vi "GrabBackground.vi"() -> ()   [LabVIEW 2011]
uses:
  <vilib>/vision/Image Controls.llb/IMAQ Image.ctl
  Main/Camera/CIGrabParams.ctl
  qtrk/QTrkLVBinding/QTrkInstance.ctl
  qtrk/QTrkLVBinding/ResultManagerInstance.ctl
  Main/Camera/CIGrabControlMsg.ctl
  Main/Camera/CIGrabControlMsgEnum.ctl
  Main/GlobalVariables.vi
  <vilib>/vision/NI_Vision_Development_Module.lvlib
panel:
  out "Image-Background":T1(plugin-control)
  in  "Export path":path
  in  "F_a":sgl=0.002
  in  "Save":bool
  out "Tmp Img":T1
  out "Background":T1(plugin-control)
  in  "Grab loop":bool
  out "Frame #":i32
  out "Image":T1(plugin-control)
  in  "Grab Framerate (Hz)":i32=20
  in  "Grab background":bool
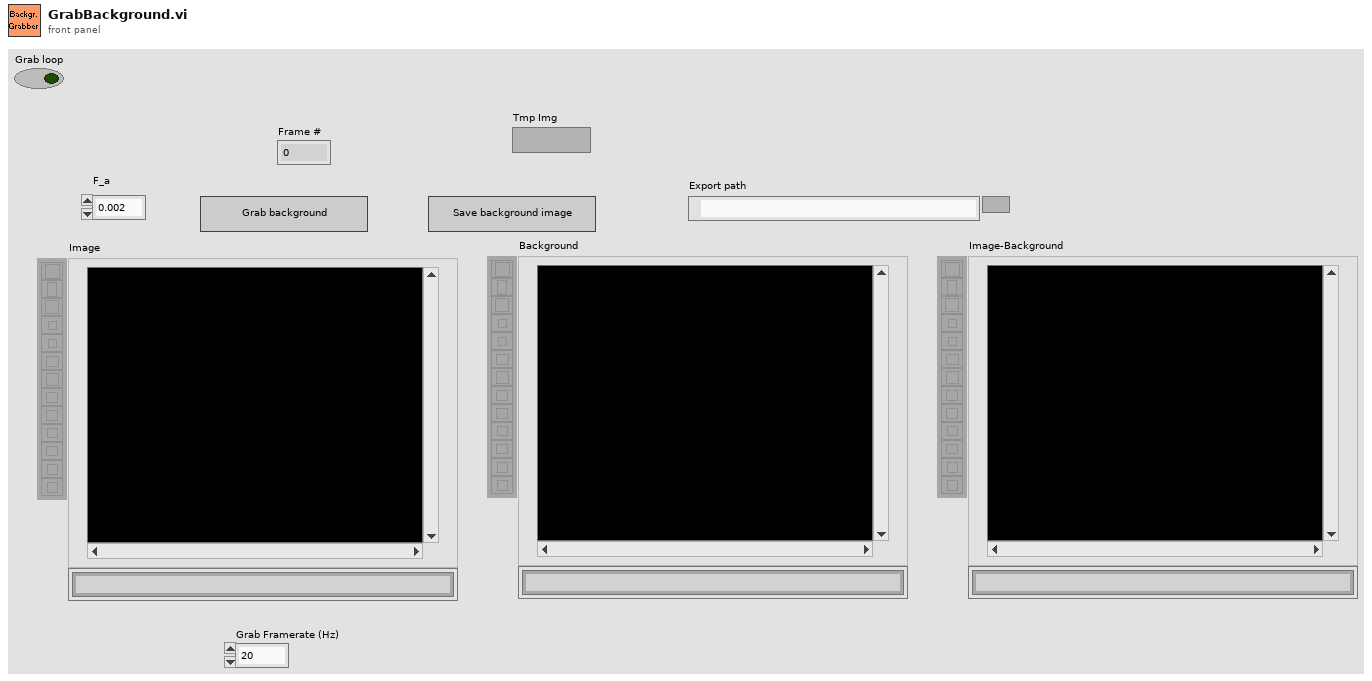
[diagram p1: front panel]
types:
  T1 = typedef "IMAQ Image.ctl" = refnum<image>
  T2 = typedef "Image Type" = u32
  T3 = enum16{"big-endian, network order", "native, host order", "little-endian"}
  T4 = typedef "CIGrabParams.ctl" = cluster{"QTrk Instance":T5, "ResultManager":T6, "Send to queue?":bool, "Force full-frame capture":bool}
  T5 = typedef "QTrkInstance.ctl" = cluster{"QTrk Pointer":u64}
  T6 = typedef "ResultManagerInstance.ctl" = cluster{"InstancePtr":u64}
  T7 = typedef "CIGrabControlMsg.ctl" = cluster{"Msg":T8}
  T8 = typedef "CIGrabControlMsgEnum.ctl" = enum16{"Stop", "EnableTracking", "DisableTracking"}
  T9 = typedef "CIGrabType.ctl" = refnum<vi>
  T10 = typedef "CmdData_NewFrame.ctl" = cluster{"Buffer Image":T1, "Frame #":i32, "Hardware ROI Index":i32, "Timestamp":dbl, "Type":T11}
  T11 = typedef "CmdEnum_CameraFrameType.ctl" = enum16{"Full", "HardwareROI", "EndGrabMarker"}
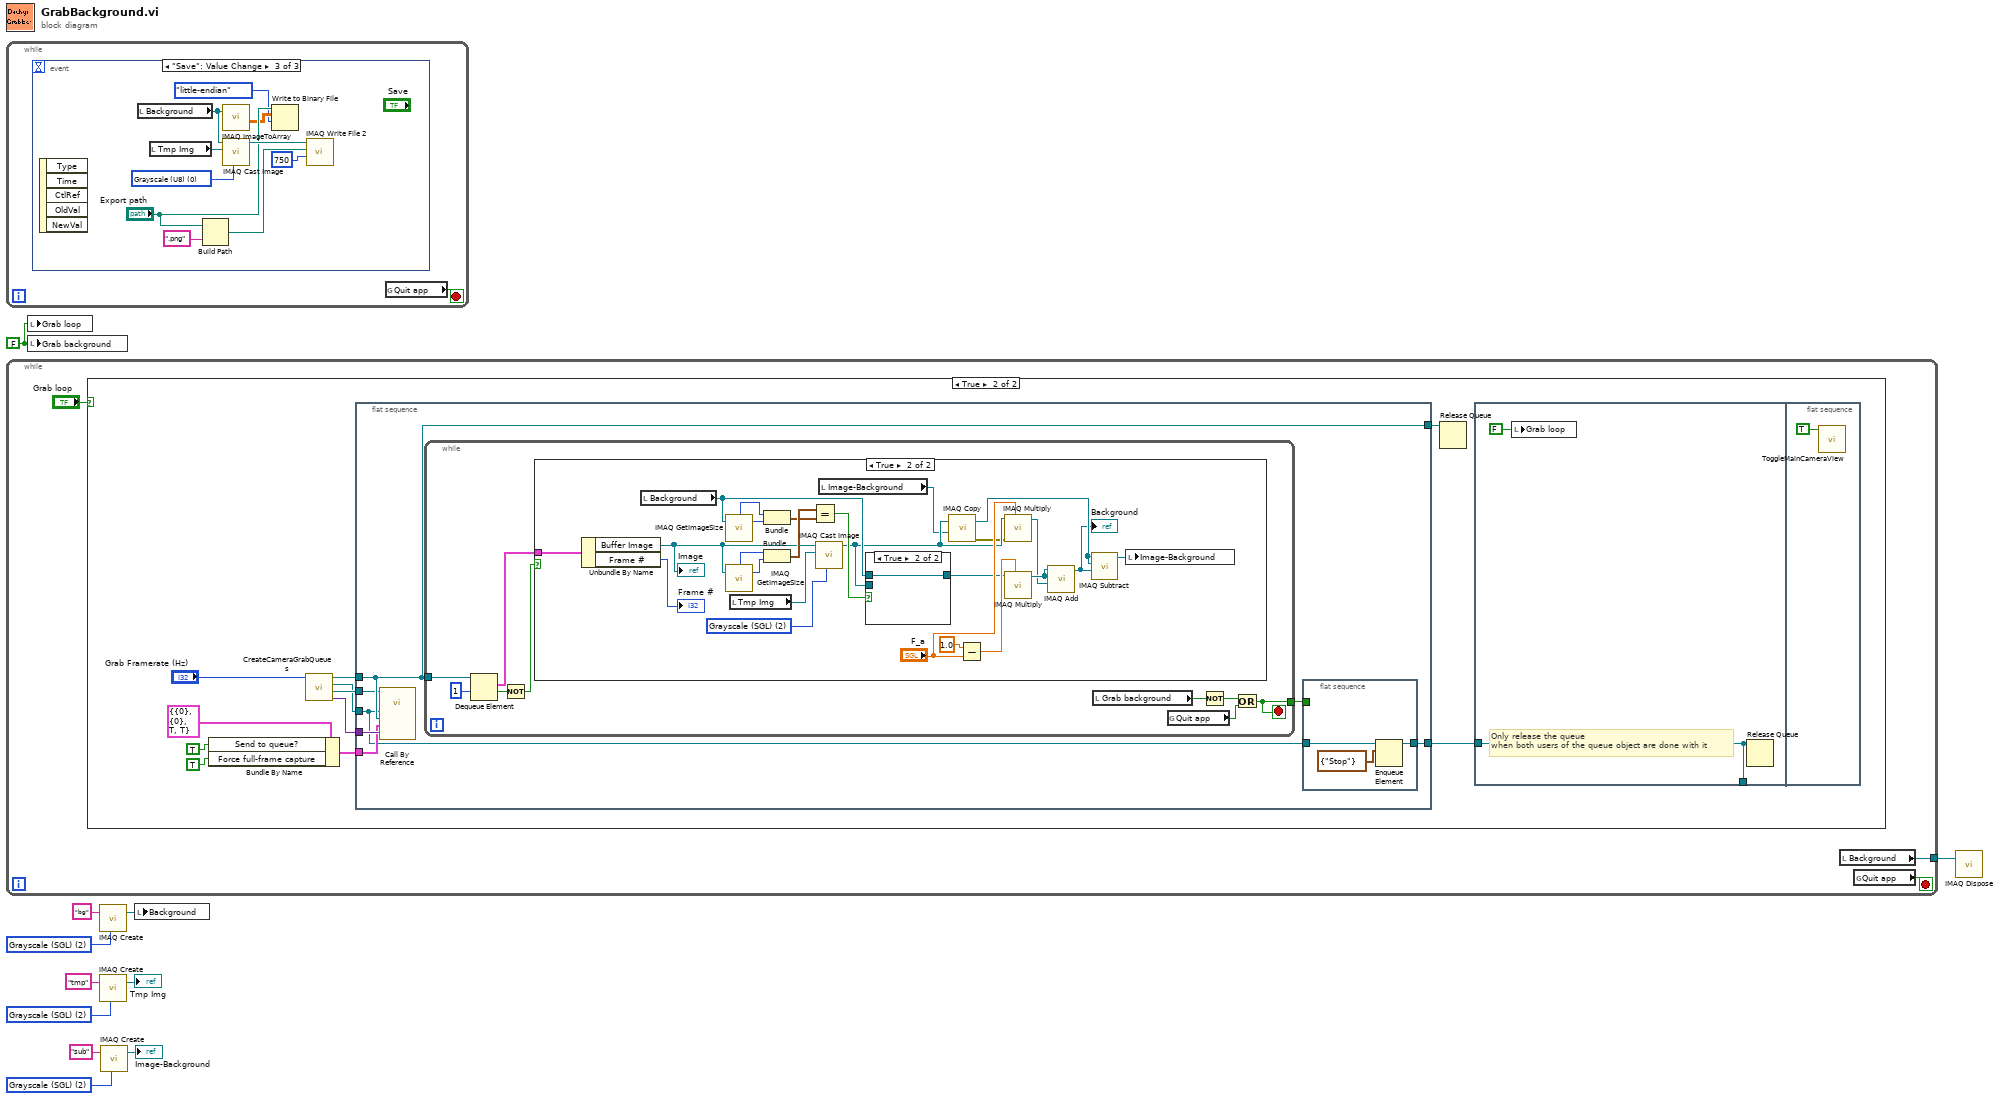
[diagram p0: block diagram]
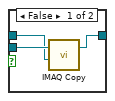
[diagram p4: hidden frame]
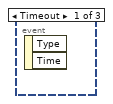
[diagram p5: hidden frame]
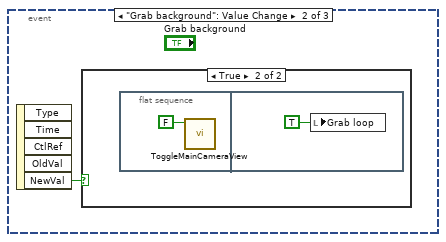
[diagram p6: hidden frame]
diagram:
  w3 = T2 2 items=["Grayscale (U8)", "Grayscale (I16)", "Grayscale (SGL)", "Complex (CSG)", "RGB (U32)", "HSL (U32)", "RGB (U64)", "Grayscale (U16)"] ("Image Type")
  w4 = T2 2 items=["Grayscale (U8)", "Grayscale (I16)", "Grayscale (SGL)", "Complex (CSG)", "RGB (U32)", "HSL (U32)", "RGB (U64)", "Grayscale (U16)"] ("Image Type")
  w5 = T2 2 items=["Grayscale (U8)", "Grayscale (I16)", "Grayscale (SGL)", "Complex (CSG)", "RGB (U32)", "HSL (U32)", "RGB (U64)", "Grayscale (U16)"] ("Image Type")
  w11 = FALSE ("Grab background")
  n1 = while {
    stop <- w12 stop-if-true
    n2 = event shown="[2] \"Save\": Value Change" {
      selector: _ -> [_ _ _]
      dyn-events: _ -> [_ _ _]
      timeout: _ -> [_ _ _]
      event Timeout {
        n3 = event-data() -> ()  [unwired: 1 in, 2 out]
      }
      event "Grab background": Value Change {
        n4 = event-data() -> ("NewVal"=w13:bool)  [unwired: 1 in, 4 out]
        n5 = case shown="True" w13 {
          frame False {
          }
          frame True {
            n6 = flat-sequence {
              frame #0 {
                n7 = call "ToggleMainCameraView.vi"("Enable? (T)"=FALSE) -> ()  [unwired: 11 in]
              }
              frame #1 {
                n8 = local write "Grab loop"(TRUE ("Grab loop")) -> ()
              }
            }
          }
        }
      }
      event "Save": Value Change {
        w22 = T2 0 items=["Grayscale (U8)", "Grayscale (I16)", "Grayscale (SGL)", "Complex (CSG)", "RGB (U32)", "HSL (U32)", "RGB (U64)", "Grayscale (U16)"] ("Image Type")
        n9 = event-data() -> ()  [unwired: 1 in, 5 out]
        n10 = local read "Background"() -> (w20:T1)
        n11 = local read "Tmp Img"() -> (w23:T1)
        n12 = Build Path(base path="Export path", name or relative path=".png") -> (appended path=w16:path)
        n13 = call "IMAQ ImageToArray"("Image"=w20) -> ("Image Pixels (Float)"=w18:sgl[][])  [unwired: 3 in, 4 out]
        n14 = call "IMAQ Cast Image"("Image Type"=w22, "Image Dst"=w23, "Image Src"=w20) -> ("Image Dst Out"=w21:T1)  [unwired: 7 in, 1 out]
        n15 = Write to Binary File(file (use dialog)="Export path", data=w18, 9:T3."little-endian" ("byte order (0:big-endian, network order)")) -> ()  [unwired: 3 in, 3 out]
        n16 = call-poly "IMAQ Write File 2"("Image Quality"=u32 750, "File Path"=w16, "Image"=w21) -> ()  [unwired: 7 in, 2 out]
      }
    }
    n17 = global read "GlobalVariables.vi" "Quit app"() -> (w12:bool)
  }
  n18 = while {
    tunnel: [w26] -> w8
    stop <- w28 stop-if-true
    n19 = case shown="True" "Grab loop" {
      frame False {
      }
      frame True {
        n20 = Bundle By Name(cluster=T4 {"QTrk Instance"={"QTrk Pointer"=0}, "ResultManager"={"InstancePtr"=0}, "Send to queue?"=TRUE, "Force full-frame capture"=TRUE} ("TrackingParameters"), "Send to queue?"=TRUE, "Force full-frame capture"=TRUE) -> (w31:T4)
        n21 = call "CreateCameraGrabQueues.vi"("Framerate (Hz)"="Grab Framerate (Hz)") -> ("Camera state (out)"=w37:variant, "VI refs.Grab"=w38:T9, "GrabControlQueue"=w30:refnum<queue>, "CameraOutQueue"=w36:refnum<queue>)  [unwired: 7 in]
        n22 = flat-sequence {
          tunnel: [w49] -> w35
          tunnel: [w48] -> w29
          tunnel: w30 -> [w43]
          tunnel: w31 -> [w45]
          tunnel: w36 -> [w49]
          tunnel: w37 -> [w46]
          tunnel: w38 -> [w47]
          frame #0 {
            n23 = call-by-ref "?"(reference=w47, "Camera data"=w46, "TrackingParameters"=w45, "Output Queue"=w49, "GrabControlQueue"=w43) -> ()  [unwired: 8 in, 3 out]
            n24 = while {
              tunnel: w49 -> [w57]
              tunnel: [w53] -> w44
              stop <- w53 stop-if-true
              n25 = Dequeue Element(queue=w57, timeout in ms (-1)=1) -> (element=w60:T10, timed out?=w59:bool)  [unwired: 1 in, 2 out]
              n26 = Not(x=w59) -> (.not. x?=w58:bool)
              n27 = case shown="True" w58 {
                tunnel: w60 -> [_ w86]
                frame False {
                }
                frame True {
                  w78 = T2 2 items=["Grayscale (U8)", "Grayscale (I16)", "Grayscale (SGL)", "Complex (CSG)", "RGB (U32)", "HSL (U32)", "RGB (U64)", "Grayscale (U16)"] ("Image Type")
                  n28 = Unbundle By Name(w86) -> ("Buffer Image"=w77:T1, "Frame #"=→"Frame #":i32)
                  "Image" <- w77
                  n29 = local read "Background"() -> (w74:T1)
                  n30 = call "IMAQ GetImageSize"("Image"=w74) -> ("Y Resolution"=w81:i32, "X Resolution"=w82:i32)  [unwired: 3 in, 1 out]
                  n31 = call "IMAQ GetImageSize"("Image"=w77) -> ("Y Resolution"=w83:i32, "X Resolution"=w84:i32)  [unwired: 3 in, 1 out]
                  n32 = local read "Tmp Img"() -> (w76:T1)
                  n33 = Bundle("X Resolution"=w82, "Y Resolution"=w81) -> (w79:cluster{"X Resolution":i32, "Y Resolution":i32})  [unwired: 1 in]
                  n34 = Bundle("X Resolution"=w84, "Y Resolution"=w83) -> (w80:cluster{"X Resolution":i32, "Y Resolution":i32})  [unwired: 1 in]
                  n35 = Equal?(x=w80, y=w79) -> (x = y?=w75:bool)
                  n36 = call "IMAQ Cast Image"("Image Type"=w78, "Image Dst"=w76, "Image Src"=w77) -> ("Image Dst Out"=w67:T1)  [unwired: 7 in, 1 out]
                  n37 = local read "Image-Background"() -> (w66:T1)
                  n38 = case shown="True" w75 {
                    tunnel: w67 -> [w89 _]
                    tunnel: w74 -> [w88 w90]
                    tunnel: [w87 w90] -> w70
                    frame False {
                      n39 = call "IMAQ Copy"("Image Dst"=w88, "Image Src"=w89) -> ("Image Dst Out"=w87:T1)  [unwired: 4 in, 1 out]
                    }
                    frame True {
                    }
                  }
                  n40 = call "IMAQ Copy"("Image Dst"=w66, "Image Src"=w67) -> ("error out"=w65:errorcluster, "Image Dst Out"=w64:T1)  [unwired: 4 in]
                  n41 = Subtract(x=1.0, y="F_a") -> (x-y=w71:dbl)
                  n42 = call "IMAQ Multiply"("Image Src A"=w67, "Constant"="F_a", "error in (no error)"=w65) -> ("Image Dst Out"=w68:T1)  [unwired: 4 in, 1 out]
                  n43 = call "IMAQ Multiply"("Image Src A"=w70, "Constant"=w71) -> ("Image Dst Out"=w69:T1)  [unwired: 5 in, 1 out]
                  n44 = call "IMAQ Add"("Image Src A"=w69, "Image Dst"=w69, "Image Src B"=w68) -> ("Image Dst Out"=w63:T1)  [unwired: 4 in, 1 out]
                  "Background" <- w63
                  n45 = call "IMAQ Subtract"("Image Src A"=w64, "Image Dst"=w64, "Image Src B"=w63) -> ("Image Dst Out"=w62:T1)  [unwired: 4 in, 1 out]
                  n46 = local write "Image-Background"(w62) -> ()
                }
              }
              n47 = local read "Grab background"() -> (w56:bool)
              n48 = global read "GlobalVariables.vi" "Quit app"() -> (w55:bool)
              n49 = Not(x=w56) -> (.not. x?=w54:bool)
              n50 = Or(x=w54, y=w55) -> (x .or. y?=w53:bool)
            }
            n51 = flat-sequence {
              tunnel: w44 -> [_]
              tunnel: w43 -> [w51]
              tunnel: [w50] -> w48
              frame #0 {
                n52 = Enqueue Element(queue=w51, element=T7 {"Msg"=enum."Stop"}) -> (queue out=w50:refnum<queue>)  [unwired: 2 in, 2 out]
              }
            }
          }
        }
        n53 = Release Queue(queue=w35) -> ()  [unwired: 2 in, 3 out]
        n54 = flat-sequence {
          tunnel: [w40] -> _
          tunnel: w29 -> [w40]
          frame #0 {
            # "Only release the queue\nwhen both users of the queue object are done with it"
            n55 = local write "Grab loop"(FALSE ("Grab loop")) -> ()
            n56 = Release Queue(queue=w40) -> ()  [unwired: 2 in, 3 out]
          }
          frame #1 {
            n57 = call "ToggleMainCameraView.vi"("Enable? (T)"=TRUE) -> ()  [unwired: 11 in]
          }
        }
      }
    }
    n58 = local read "Background"() -> (w26:T1)
    n59 = global read "GlobalVariables.vi" "Quit app"() -> (w28:bool)
  }
  n60 = local write "Grab loop"(w11) -> ()
  n61 = local write "Grab background"(w11) -> ()
  n62 = call "IMAQ Create"("Image Name"="bg", "Image Type"=w4) -> ("New Image"=w10:T1)  [unwired: 3 in, 1 out]
  n63 = call "IMAQ Create"("Image Name"="tmp", "Image Type"=w5) -> ("New Image"=→"Tmp Img":T1)  [unwired: 3 in, 1 out]
  n64 = call "IMAQ Create"("Image Name"="sub", "Image Type"=w3) -> ("New Image"=→"Image-Background":T1)  [unwired: 3 in, 1 out]
  n65 = local write "Background"(w10) -> ()
  n66 = call "IMAQ Dispose"("Image"=w8) -> ()  [unwired: 5 in, 1 out]
